vi "MongoDB.DropCollection.vi"(8 "error in (no error)":errorcluster, 10 "collectionName":string, 11 "MongoDB.Database in":refnum<class "MongoDB.Database.lvclass">) -> (0 "error out":errorcluster, 3 "MongoDB.Database out":refnum<class "MongoDB.Database.lvclass">)   [LabVIEW 2014, in "MongoDB.Database.lvclass"]
uses:
  MongoDB.Database.lvclass
  MongoDB.Database.lvclass/MongoDB.Database.ctl
  C:/Users/Richard/Documents/GitHub/mongo-labview-driver/CSharp/bin/MongoDB.Driver.Legacy.dll
  CSharp/bin/MongoDB.Driver.Legacy.dll
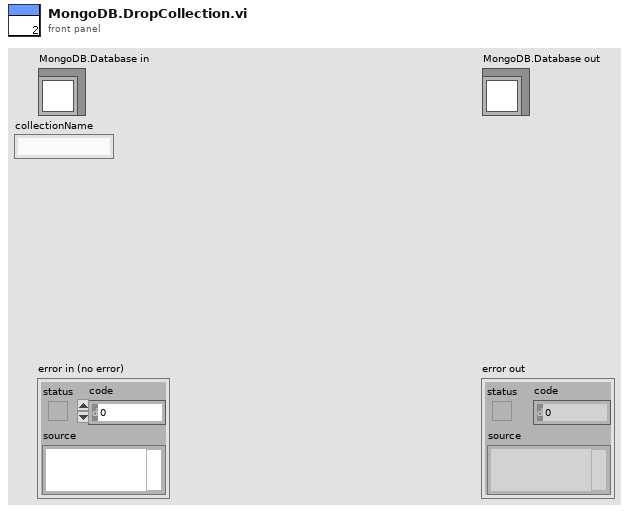
[diagram p1: front panel]
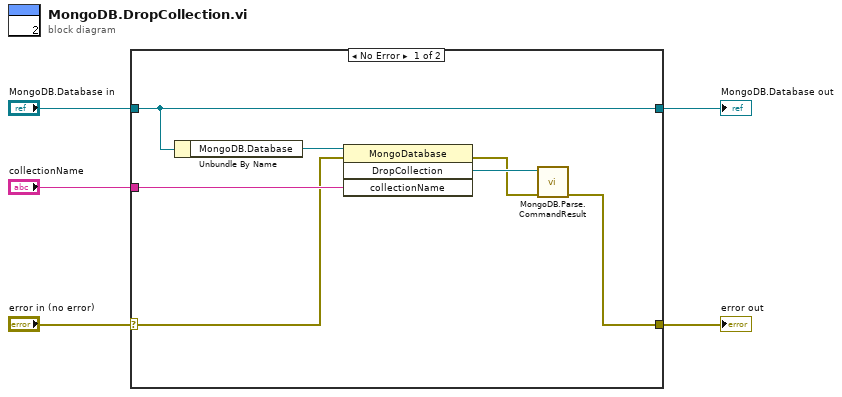
[diagram p0: block diagram]
diagram:
  n1 = case shown="No Error" "error in (no error)" {
    selector: "error in (no error)" -> [w7 w14]
    tunnel: [w6 w14] -> w4
    tunnel: [w12 w13] -> w2
    tunnel: "MongoDB.Database in" -> [w12 w13]
    tunnel: "collectionName" -> [w10 _]
    frame No Error {
      n2 = Unbundle By Name(w12) -> ("MongoDB.Database"=w11:refnum<k24>)
      n3 = invoke class="MongoDatabase" method="DropCollection"(reference=w11, error in=w7, "collectionName"=w10) -> (error out=w8:errorcluster, "DropCollection"=w9:refnum<k24>)  [unwired: 1 in, 2 out]
      n4 = call "MongoDB.Parse.CommandResult.vi"("error in (no error)"=w8, "MongoDB.Command.Result"=w9) -> ("error out"=w6:errorcluster)  [unwired: 9 in]
    }
    frame Error {
    }
  }
  "error out" <- w4
  "MongoDB.Database out" <- w2
